vi "e.gate Count Time Elements.vi"(8 "error in (no error)":errorcluster, 11 "Time Format String":string) -> (0 "error out":cluster{"status":bool, i32, "source":string}, 3 "NumberOfTimeElements":i32)   [LabVIEW 2016]
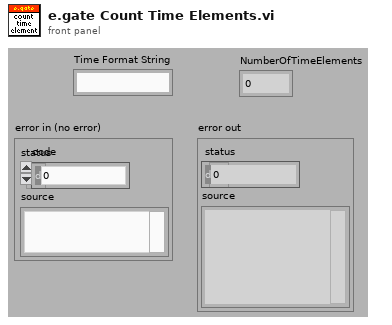
[diagram p1: front panel]
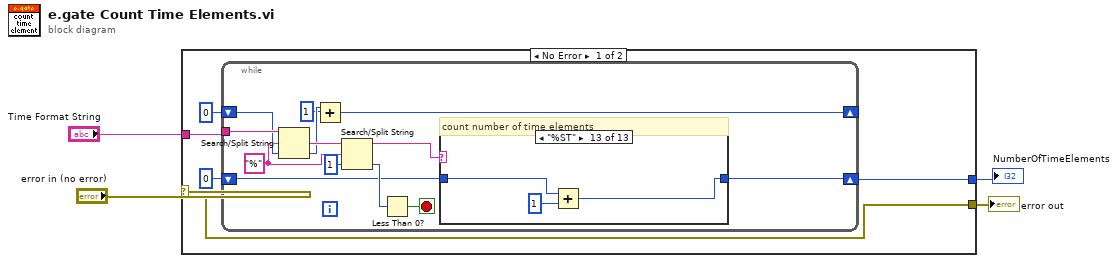
[diagram p0: block diagram]
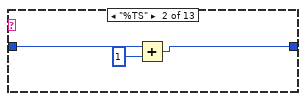
[diagram p3: hidden frame]
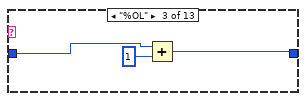
[diagram p4: hidden frame]
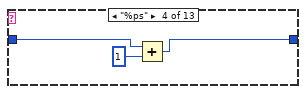
[diagram p5: hidden frame]
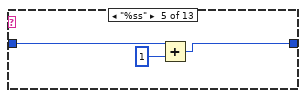
[diagram p6: hidden frame]
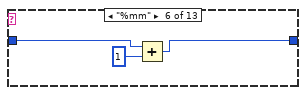
[diagram p7: hidden frame]
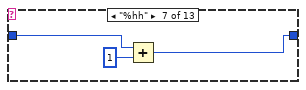
[diagram p8: hidden frame]
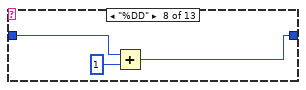
[diagram p9: hidden frame]
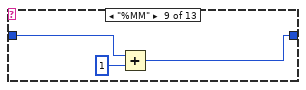
[diagram p10: hidden frame]
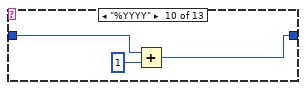
[diagram p11: hidden frame]
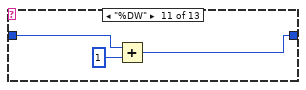
[diagram p12: hidden frame]
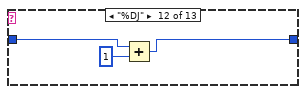
[diagram p13: hidden frame]
diagram:
  n1 = case shown="No Error" "error in (no error)" {
    selector: "error in (no error)" -> [w7 w60]
    tunnel: [w7 w60] -> w3
    tunnel: "Time Format String" -> [w9 _]
    tunnel: [w5 _] -> w1
    frame No Error {
      n2 = while {
        tunnel: w9 -> [w22]
        shift-right: [w14] -> _
        shift-left: 0 -> [w21]
        shift-right: [w10] -> w5
        shift-left: 0 -> [w11]
        stop <- w16 stop-if-true
        w18 = "%" ("Nach String/Zeichen suchen (-)")
        # "count number of time elements"
        n3 = Search/Split String(string=w22, search string/char (-)=w18, offset (0)=w21) -> (match + rest of string=w20:string, offset of match=w13:i32)  [unwired: 1 out]
        n4 = Add ("Addieren")(x=w13, y=1) -> (x+y=w14:i32)
        n5 = Search/Split String(string=w20, search string/char (-)=w18, offset (0)=1 ("Offset (0)")) -> (substring before match=w17:string, offset of match=w15:i32)  [unwired: 1 out]
        n6 = Less Than 0?(x=w15) -> (x < 0?=w16:bool)
        n7 = case shown="\"%ST\"" w17 {
          tunnel: w11 -> [w23 w26 w28 w31 w34 w37 w40 w43 w46 w49 w52 w55 w58]
          tunnel: [w23 w25 w27 w30 w33 w36 w39 w42 w45 w48 w51 w54 w57] -> w10
          frame "", Default {
          }
          frame "%TS" {
            n8 = Add(x=w26, y=1) -> (x+y=w25:i32)
          }
          frame "%OL" {
            n9 = Add(x=w28, y=1) -> (x+y=w27:i32)
          }
          frame "%ps" {
            n10 = Add(x=w31, y=1) -> (x+y=w30:i32)
          }
          frame "%ss" {
            n11 = Add(x=w34, y=1) -> (x+y=w33:i32)
          }
          frame "%mm" {
            n12 = Add(x=w37, y=1) -> (x+y=w36:i32)
          }
          frame "%hh" {
            n13 = Add(x=w40, y=1) -> (x+y=w39:i32)
          }
          frame "%DD" {
            n14 = Add(x=w43, y=1) -> (x+y=w42:i32)
          }
          frame "%MM" {
            n15 = Add(x=w46, y=1) -> (x+y=w45:i32)
          }
          frame "%YYYY" {
            n16 = Add(x=w49, y=1) -> (x+y=w48:i32)
          }
          frame "%DW" {
            n17 = Add(x=w52, y=1) -> (x+y=w51:i32)
          }
          frame "%DJ" {
            n18 = Add(x=w55, y=1) -> (x+y=w54:i32)
          }
          frame "%ST" {
            n19 = Add(x=w58, y=1) -> (x+y=w57:i32)
          }
        }
      }
    }
    frame Error {
    }
  }
  "error out" <- w3
  "NumberOfTimeElements" <- w1
